vi "Parse Close Delimiter.vi"(8 "Error In":errorcluster, 11 "Parser In":refnum<class "Parser.lvclass">) -> (0 "Error Out":errorcluster, 3 "Parser Out":refnum<class "Parser.lvclass">)   [LabVIEW 2017, in "Mustache.lvlib" / "Parser.lvclass"]
uses:
  Parser.lvclass
  Parser.lvclass/Parser.ctl
  Public/Controls/States.ctl
  Tokens/Public/EscapedVariable/EscapedVariable.lvclass
  D:/Users/cfield/Code/Field R&D Services/Mustache/feature-lv-original-parser/src/Mustache/Public/Tokens/Public/Abstract/Abstract.lvclass
  Tokens/Public/UnescapedVariable/UnescapedVariable.lvclass
  Tokens/Public/BeginSection/BeginSection.lvclass
  Tokens/Public/InvertedSection/InvertedSection.lvclass
  Tokens/Public/EndSection/EndSection.lvclass
  Tokens/Public/EndSection/Public/New.vi
  Tokens/Public/InvertedSection/Public/New.vi
  Tokens/Public/BeginSection/Public/New.vi
  Tokens/Public/UnescapedVariable/Public/New.vi
  Tokens/Public/EscapedVariable/Public/New.vi
  <vilib>/Utility/error.llb/Trim Whitespace.vi
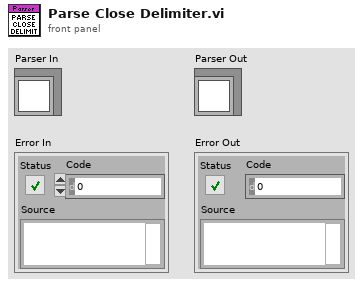
[diagram p1: front panel]
types:
  T1 = typedef "Mustache.lvlib/Parser.lvclass/States.ctl" = enum16{"Text", "Open Delimiter", "Tag Type", "Tag Key", "Close Delimiter"}
  T2 = typedef "Mustache.lvlib/Parser.lvclass/Tag Types.ctl" = enum16{"Escaped Variable", "{} Unescaped Variable", "& Unescaped Variable", "Begin Section", "Inverted Section", "End Section", "Comment", "Partial", "Set Delimiter"}
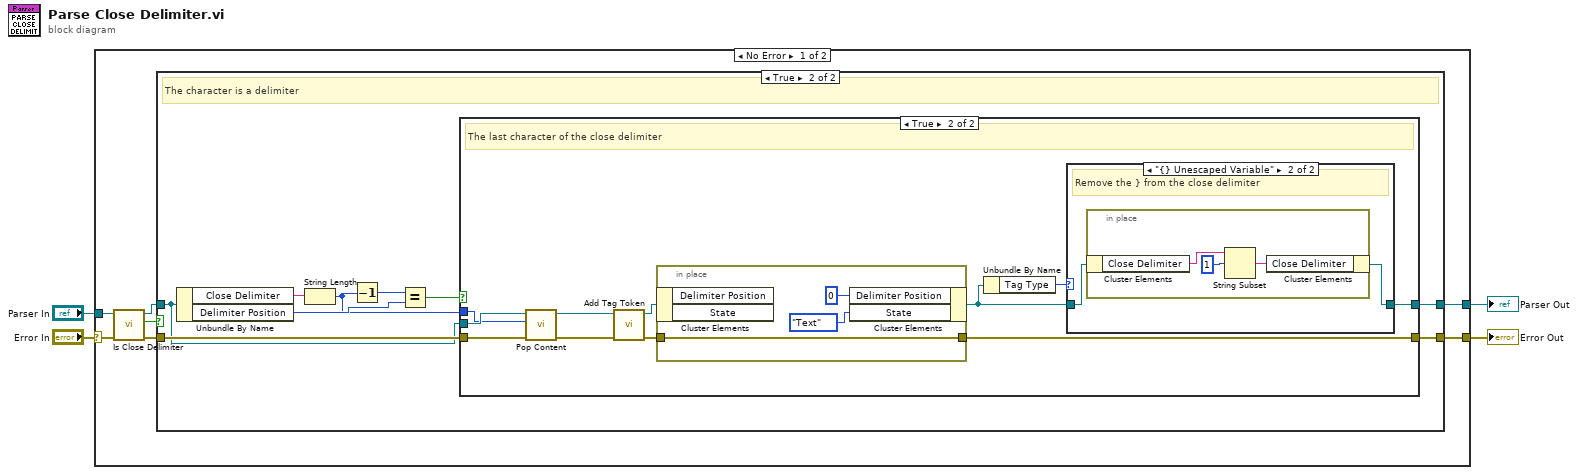
[diagram p0: block diagram]
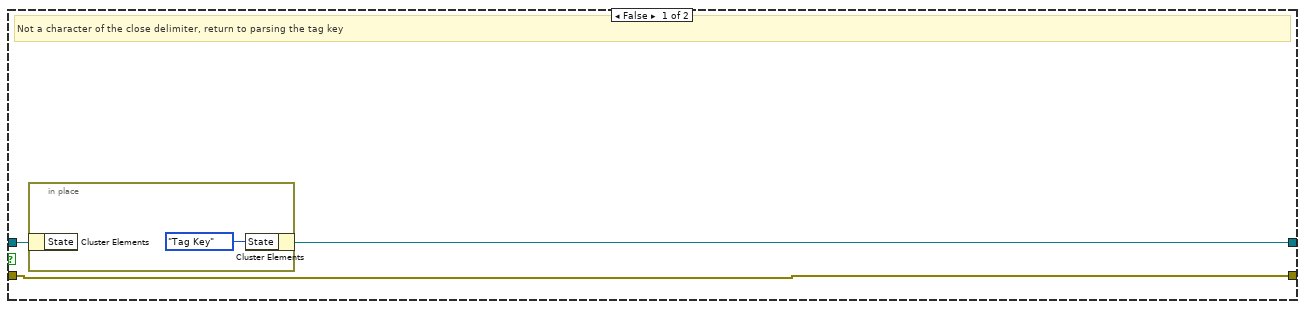
[diagram p2: hidden frame]
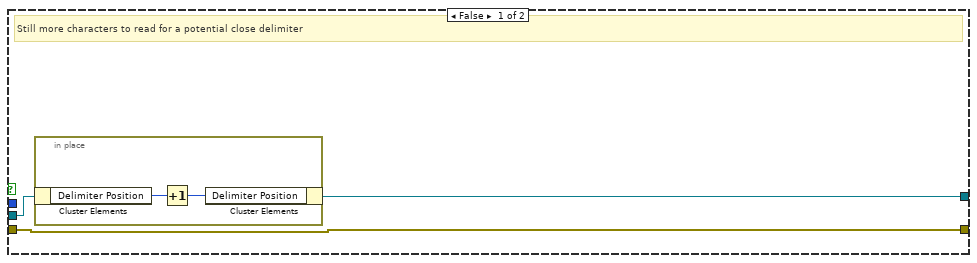
[diagram p3: hidden frame]
diagram:
  n1 = case shown="No Error" "Error In" {
    selector: "Error In" -> [w10 w50]
    tunnel: [w6 w50] -> w4
    tunnel: [w5 w51] -> w3
    tunnel: "Parser In" -> [w11 w51]
    frame No Error {
      n2 = call "Is Close Delimiter.vi"("Error In"=w10, "Parser In"=w11) -> ("Error Out"=w9:errorcluster, "Close Delimiter"=w7:bool, "Parser Out"=w8:refnum<class "Parser.lvclass">)  [unwired: 7 in]
      n3 = case shown="True" w7 {
        tunnel: w9 -> [w14 w21]
        tunnel: w8 -> [w13 w20]
        tunnel: [w14 w18] -> w6
        tunnel: [w12 w19] -> w5
        frame False {
          # "Not a character of the close delimiter, return to parsing the tag key"
          n4 = in-place {
            n5 = in-place-cluster #1(w13) -> ()  [unwired: 1 out]
            n6 = in-place-cluster #1("State"=States."Tag Key") -> (w12:refnum<class "Parser.lvclass">)
          }
        }
        frame True {
          # "The character is a delimiter"
          n7 = Unbundle By Name(w20) -> ("Close Delimiter"=w17:string, "Delimiter Position"=w23:i32)
          n8 = String Length(string=w17) -> (length=w16:i32)
          n9 = Decrement(x=w16) -> (x-1=w24:i32)
          n10 = Equal?(x=w24, y=w23) -> (x = y?=w22:bool)
          n11 = case shown="True" w22 {
            tunnel: w21 -> [w25 w40]
            tunnel: w20 -> [w27 w35]
            tunnel: [w26 w30] -> w19
            tunnel: [w25 w36] -> w18
            tunnel: w16 -> [_ w33]
            frame False {
              # "Still more characters to read for a potential close delimiter"
              n12 = in-place {
                n13 = in-place-cluster #2(w27) -> ("Delimiter Position"=w29:i32)
                n14 = Increment(x=w29) -> (x+1=w28:i32)
                n15 = in-place-cluster #2("Delimiter Position"=w28) -> (w26:refnum<class "Parser.lvclass">)
              }
            }
            frame True {
              # "The last character of the close delimiter"
              n16 = call "Pop Content.vi"("Error In"=w40, "Characters Count"=w33, "Parser In"=w35) -> ("Error Out"=w34:errorcluster, "Parser Out"=w39:refnum<class "Parser.lvclass">)  [unwired: 7 in]
              n17 = call "Add Tag Token.vi"("Error In"=w34, "Parser In"=w39) -> ("Error Out"=w37:errorcluster, "Parser Out"=w38:refnum<class "Parser.lvclass">)  [unwired: 8 in]
              n18 = in-place {
                in-place-border: w37 -> [w49]
                in-place-border: [w49] -> w36
                n19 = in-place-cluster #3(w38) -> ()  [unwired: 2 out]
                n20 = in-place-cluster #3("Delimiter Position"=0, "State"=States."Text") -> (w31:refnum<class "Parser.lvclass">)
              }
              n21 = Unbundle By Name(w31) -> ("Tag Type"=w32:T2)
              n22 = case shown="\"{} Unescaped Variable\"" w32 {
                tunnel: w31 -> [w41 w43]
                tunnel: [w41 w42] -> w30
                frame "Escaped Variable", Default {
                }
                frame "{} Unescaped Variable" {
                  # "Remove the } from the close delimiter"
                  n23 = in-place {
                    n24 = in-place-cluster #4(w43) -> ("Close Delimiter"=w46:string)
                    n25 = String Subset(string=w46, offset (0)=1) -> (substring=w44:string)  [unwired: 1 in]
                    n26 = in-place-cluster #4("Close Delimiter"=w44) -> (w42:refnum<class "Parser.lvclass">)
                  }
                }
              }
            }
          }
        }
      }
    }
    frame Error {
    }
  }
  "Error Out" <- w4
  "Parser Out" <- w3
